vi "FiberSpectrograph_logEvent_rejectedCommand.vi"(8 "error in (no error)":errorcluster, 11 "logevent_rejectedCommand_Ctl":T1) -> (0 "error out":errorcluster, 2 "function return":i32, 3 "logevent_rejectedCommand_Ctl out":T1)   [LabVIEW 2016, in "SALLV_FiberSpectrograph.lvlib"]
doc: "int FiberSpectrograph_shm_logEvent_rejectedCommandLV(FiberSpectrograph_logevent_rejectedCommandLV *logevent_rejectedCommand_Ctl );"
uses:
  SALLV_FiberSpectrograph.lvlib
  DataTypes/logevent_rejectedCommand.ctl
  SALLV_FiberSpectrograph.so
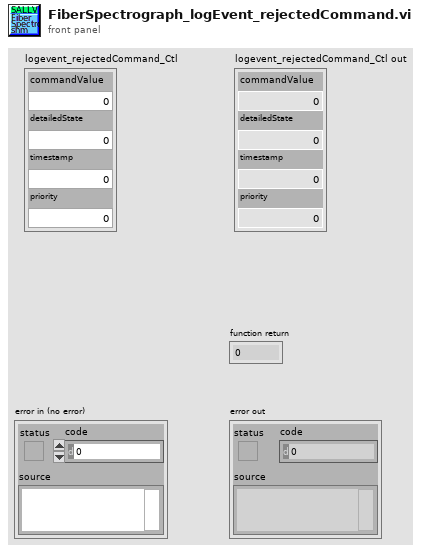
[diagram p1: front panel]
types:
  T1 = typedef "SALLV_FiberSpectrograph.lvlib/logevent_rejectedCommand.ctl" = cluster{"commandValue":u16, "detailedState":u16, "timestamp":dbl, "priority":i32}
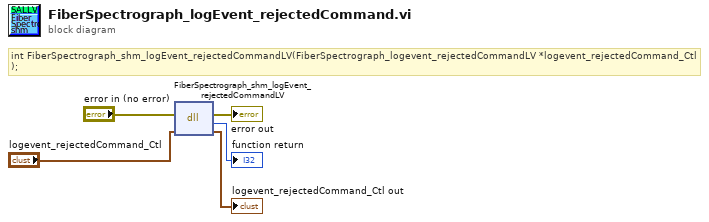
[diagram p0: block diagram]
diagram:
  # "int FiberSpectrograph_shm_logEvent_rejectedCommandLV(FiberSpectrograph_logevent_rejectedCommandLV *logevent_rejectedCommand_Ctl );"
  n1 = dll-call lib="home/harini/Documents/lsst/SALLV_FiberSpectrograph/SALLV_FiberSpectrograph.*" fn="FiberSpectrograph_shm_logEvent_rejectedCommandLV"(error in="error in (no error)", "logevent_rejectedCommand_Ctl"="logevent_rejectedCommand_Ctl") -> (error out=→"error out":errorcluster, →"function return":i32, "logevent_rejectedCommand_Ctl"=→"logevent_rejectedCommand_Ctl out":T1)  [unwired: 2 in, 1 out]
